vi "PCIe SLM - Startup.vi"(8 "error in (no error)":errorcluster, 11 "LUT Path":path=path "D:/Software/Optical-Prime/Instruments/SLM/LUT.lut") -> (0 "error out":errorcluster, 2 "SLM Params":T1={"Width"=1920.0, "Height"=1152.0, "Board ID"=1, "Centre Y"=0.462, "Centre X"=0.386} {"Centre X" format="%.3g"; "Centre Y" format="%.3g"}, 3 "LUT_file out":path=path "D:/Software/Optical-Prime/Instruments/SLM/LUT.lut")   [LabVIEW 2020]
uses:
  _controls/PCIe SLM params.ctl
  <userlib>/SLM Lib/SLM Lib.lvlib
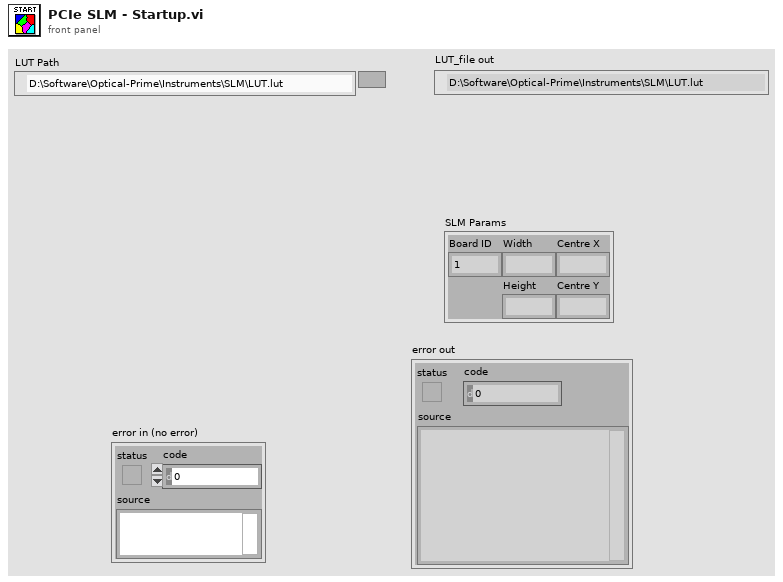
[diagram p1: front panel]
types:
  T1 = typedef "PCIe SLM params.ctl" = cluster{"Width":dbl, "Height":dbl, "Board ID":i32, "Centre Y":dbl, "Centre X":dbl}
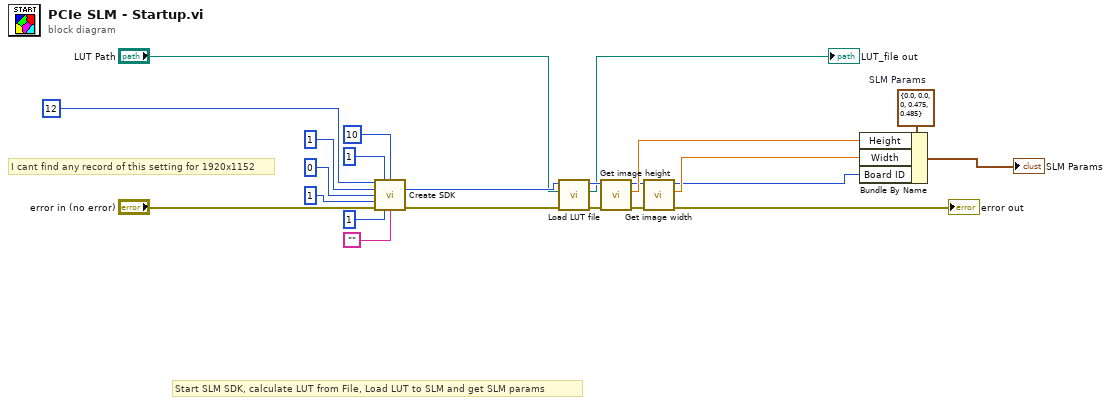
[diagram p0: block diagram]
diagram:
  w3 = T1 {"Width"=0.0, "Height"=0.0, "Board ID"=0, "Centre Y"=0.475, "Centre X"=0.485}  # SLM Params
  # "I cant find any record of this setting for 1920x1152"
  # "Start SLM SDK, calculate LUT from File, Load LUT to SLM and get SLM params"
  n1 = call <userlib>:"Create SDK.vi"("SLM_bit_depth"=u32 12, "RAM_write_enable"=1, "max_transient_frames"=10, "n_boards_found"=u32 1, "constructed_ok"=0, "is_nematic_type"=1, "error in (no error)"="error in (no error)", "use_GPU_if_available"=1, "static_regional_lut_file"="") -> ("n_boards_found out"=w22:i32, "error out"=w8:errorcluster)  [unwired: 3 in, 2 out]
  n2 = call <userlib>:"Load LUT file.vi"("error in (no error)"=w8, "LUT_file"="LUT Path", "board IN"=w22) -> ("error out"=w23:errorcluster, "LUT_file out"=→"LUT_file out":path, "board OUT"=w14:i32)  [unwired: 6 in]
  n3 = call <userlib>:"Get image height.vi"("error in (no error)"=w23, "board IN"=w14) -> ("error out"=w21:errorcluster, "Height"=w13:dbl, "board OUT"=w12:i32)  [unwired: 7 in]
  n4 = call <userlib>:"Get image width.vi"("error in (no error)"=w21, "board IN"=w12) -> ("error out"=→"error out":errorcluster, "Width"=w11:dbl, "board OUT"=w1:i32)  [unwired: 7 in]
  n5 = Bundle By Name(cluster=w3, "Height"=w13, "Width"=w11, "Board ID"=w1) -> (→"SLM Params":T1)
